vi "ExSubNframeColQ.vi"(2 "error in (no error)":errorcluster, 3 "Number of Images":u32=1 min=1 step=1, 4 "Handle Cluster":T1) -> (0 "error out":errorcluster, 1 "Handle Cluster":T1)   [LabVIEW 2010]
panel:
  # "ExSubNframeColCoolSnap:\nThis is a sub VI that collects N frames from the camera\nsystem. This assumes camera has been setup and \ninitialized and that the start camera is done. It also \nassumes the camera has circular buffer capabillities.\nThis is not true for all cameras, especially older \nPhotometrics cameras."
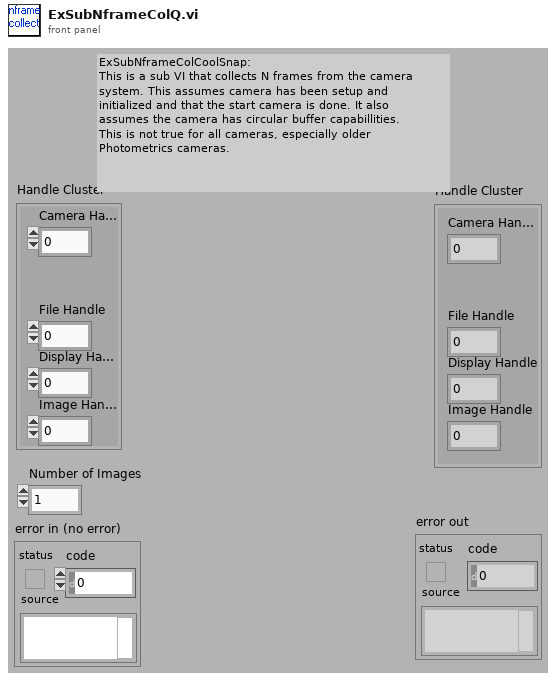
[diagram p1: front panel]
types:
  T1 = cluster{"Camera Handle":u32, "File Handle":u32, "Display Handle":u32, "Image Handle":u32}
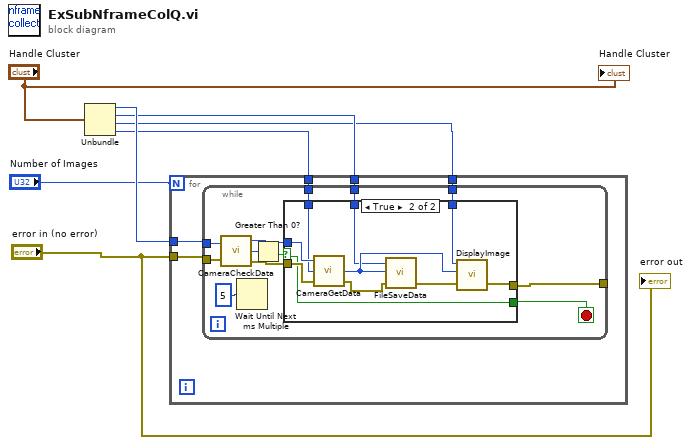
[diagram p0: block diagram]
diagram:
  n1 = Unbundle("Handle Cluster") -> ("Camera Handle"=w7:u32, "File Handle"=w3:u32, "Display Handle"=w2:u32, "Image Handle"=w1:u32)
  n2 = for {
    N: "Number of Images" -> [_]
    tunnel: w7 -> [w12]
    tunnel: w3 -> [w11]
    tunnel: w2 -> [w10]
    tunnel: w1 -> [w9]
    tunnel: "error in (no error)" -> [w8]
    n3 = while {
      tunnel: w8 -> [w23]
      tunnel: w12 -> [w22]
      tunnel: [w17] -> _
      tunnel: w11 -> [w16]
      tunnel: w10 -> [w15]
      tunnel: w9 -> [w14]
      stop <- w18 stop-if-true
      n4 = call <userlib>:"CameraCheckData.vi"("Camera Handle"=w22, "error in"=w23) -> ("Camera Handle"=w20:u32, "Number Of Frames Available"=w24:i32, "error out"=w19:errorcluster)
      n5 = Wait Until Next ms Multiple(millisecond multiple=5) -> ()  [unwired: 1 out]
      n6 = Greater Than 0?(x=w24) -> (x > 0?=w21:bool)
      n7 = case shown="True" w21 {
        selector: w21 -> [w25 w34]
        tunnel: w20 -> [_ w36]
        tunnel: w19 -> [w26 w35]
        tunnel: [w25 w34] -> w18
        tunnel: [w26 w31] -> w17
        tunnel: w16 -> [_ w29]
        tunnel: w15 -> [_ w28]
        tunnel: w14 -> [_ w27]
        frame False {
        }
        frame True {
          n8 = call <userlib>:"CameraGetData.vi"("error in"=w35, "Data Handle"=w27, "Camera Handle"=w36) -> ("error out"=w33:errorcluster, "Data Handle"=w30:u32)  [unwired: 1 out]
          n9 = call <userlib>:"FileSaveData.vi"("error in"=w33, "Image Handle"=w30, "File Handle"=w29) -> ("error out"=w32:errorcluster)  [unwired: 1 out]
          n10 = call <userlib>:"DisplayImage.vi"("error in"=w32, "Image Handle"=w30, "Display Handle"=w28) -> ("error out"=w31:errorcluster)  [unwired: 1 in, 1 out]
        }
      }
    }
  }
  "error out" <- "error in (no error)"
  "Handle Cluster" <- "Handle Cluster"
